vi "Configure Trigger.vi"(8 "error in (no error)":errorcluster, 10 "Trigger Source (0:Manual)":i32(ring) items=["Manual", "Bus"], 11 "VISA resource name":refnum<visa-resource-name>) -> (0 "error out":errorcluster, 3 "VISA resource name out":refnum<visa-resource-name>)   [LabVIEW 2021, in "BK Precision 9200 Series.lvlib"]
doc: "Configures the trigger source. Trigger is used to initiate the start of a list program."
uses:
  <instrlib>/BK Precision 9200 Series/BK Precision 9200 Series.lvlib
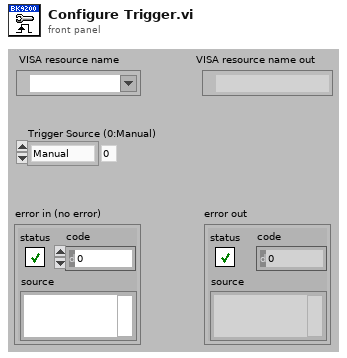
[diagram p1: front panel]
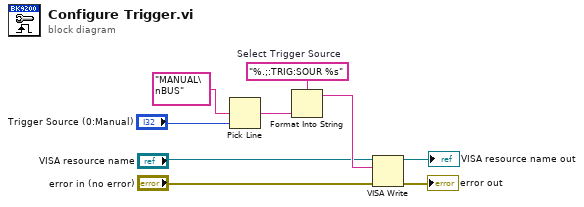
[diagram p0: block diagram]
diagram:
  w9 = "%.;:TRIG:SOUR %s"  # Select Trigger Source
  n1 = Pick Line(multi-line string="MANUAL\nBUS", line index="Trigger Source (0:Manual)") -> (output string=w7:string)  [unwired: 1 in]
  n2 = Format Into String(format string=w9, w7) -> (resulting string=w5:string)  [unwired: 2 in, 1 out]
  n3 = VISA Write(VISA resource name="VISA resource name", write buffer=w5, error in (no error)="error in (no error)") -> (VISA resource name out=→"VISA resource name out":refnum<visa-resource-name>, error out=→"error out":errorcluster)  [unwired: 1 out]
